vi "LogAddLine.vi"(7 "error in (no error)":errorcluster, 9 "Msg in":string, 10 "String in":refnum<vi>) -> (0 "error out":errorcluster, 3 "String out":refnum<vi>)   [LabVIEW 2017]
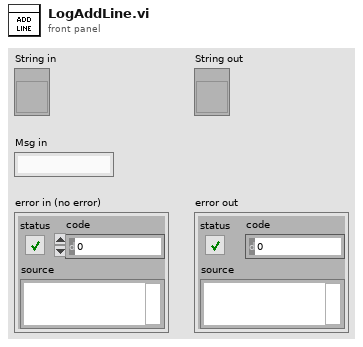
[diagram p1: front panel]
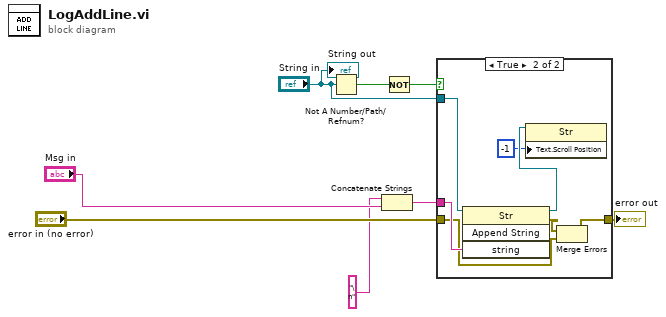
[diagram p0: block diagram]
diagram:
  n1 = Not A Number/Path/Refnum?(number/path/refnum="String in") -> (NaN/Path/Refnum?=w3:bool)
  n2 = Concatenate Strings("\n" ("string"), "Msg in") -> (w5:string)
  n3 = Not(x=w3) -> (.not. x?=w2:bool)
  n4 = case shown="True" w2 {
    tunnel: w5 -> [_ w16]
    tunnel: "error in (no error)" -> [w9 w12]
    tunnel: [w9 w13] -> w4
    tunnel: "String in" -> [_ w15]
    frame False {
    }
    frame True {
      n5 = invoke class="Str" method="Append String"(reference=w15, "string"=w16) -> (reference out=w11:refnum<vi>, error out=w14:errorcluster)  [unwired: 2 in, 2 out]
      n6 = property class="Str"(reference=w11, "Text.Scroll Position"=-1) -> ()  [unwired: 1 in, 2 out]
      n7 = Merge Errors(w14, w12) -> (w13:errorcluster)
    }
  }
  "error out" <- w4
  "String out" <- "String in"
